vi "normal.vi"(3 "Settings":T1={"Horizontal Conf."={"Min. Sample rate"=0.0, "Reference position"=0.0, "Record Length"=0}, "Channel A"={"Enable"=FALSE, "Vertical coupling"=0, "Vertical range"=0.0, "Vertical offset"=0.0, "Probe attenuation"=1.0}, "Channel B"={"Enable"=FALSE, "Vertical coupling"=0, "Vertical range"=0.0, "Vertical offset"=0.0, "Probe attenuation"=1.0}, "Trigger"={"Source"=enum."channel 1", "Slope"=enum."Positive", "Coupling"=enum."AC", "Level"=0.0, "Holdoff"=0.0, "Delay"=0.0, "Timeout"=0.0, "Mode"=enum."Normal"}, "Measurements"={"Measurement 1, Channel"=enum."Channel 1", "Measurement 1, Selection"=enum."", "Measurement 2, Channel"=enum."Channel 1", "Measurement 2,  Selection"=enum."", "Measurement 3, Channel"=enum."Channel 1", "Measurement 3, Selection 3"=enum.""}}, 4 "error in":errorcluster caption="Error in" {"code" format="%.0x"}, 5 "instrument handle in":refnum<k15>) -> (0 "error out":errorcluster caption="Error out" {"code" format="%.0x"}, 1 "Adjusted Trigger Level":dbl, 2 "instrument handle out":refnum<k15>)   [LabVIEW 2011]
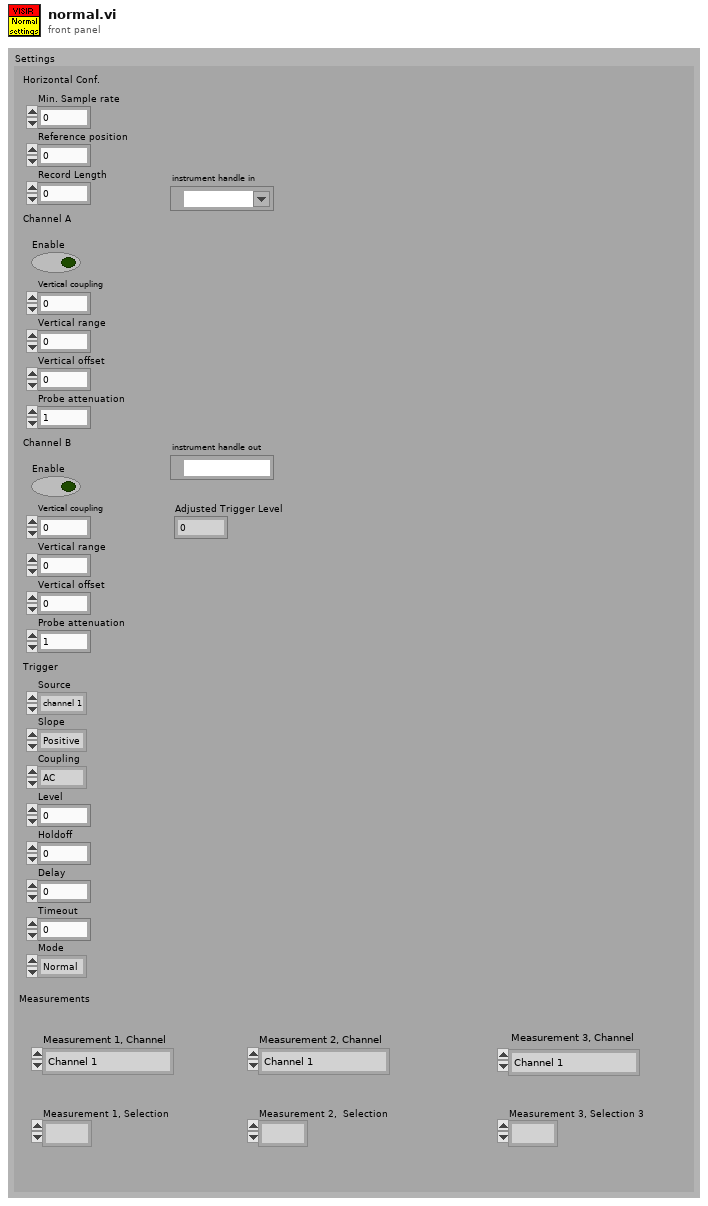
[diagram p1: front panel]
types:
  T1 = cluster{"Horizontal Conf.":cluster{"Min. Sample rate":dbl, "Reference position":dbl, "Record Length":i16}, "Channel A":cluster{"Enable":bool, "Vertical coupling":i32, "Vertical range":dbl, "Vertical offset":dbl, "Probe attenuation":dbl}, "Channel B":cluster{"Enable":bool, "Vertical coupling":i32, "Vertical range":dbl, "Vertical offset":dbl, "Probe attenuation":dbl}, "Trigger":cluster{"Source":enum8{"channel 1", "channel 2", "Imediate", "External trigger"}, "Slope":enum8{"Positive", "Negative"}, "Coupling":enum8{"AC", "DC"}, "Level":dbl, "Holdoff":dbl, "Delay":dbl, "Timeout":dbl, "Mode":enum8{"Normal", "Auto", "Auto Level"}}, "Measurements":cluster{"Measurement 1, Channel":enum8{"Channel 1", "Channel 2", "Channel 3", "Channel 4"}, "Measurement 1, Selection":enum16{""}, "Measurement 2, Channel":enum8{"Channel 1", "Channel 2", "Channel 3", "Channel 4"}, "Measurement 2,  Selection":enum16{""}, "Measurement 3, Channel":enum8{"Channel 1", "Channel 2", "Channel 3", "Channel 4"}, "Measurement 3, Selection 3":enum16{""}}}
  T2 = cluster{"Min. Sample rate":dbl, "Reference position":dbl, "Record Length":i16}
  T3 = cluster{"Enable":bool, "Vertical coupling":i32, "Vertical range":dbl, "Vertical offset":dbl, "Probe attenuation":dbl}
  T4 = cluster{"Source":enum8{"channel 1", "channel 2", "Imediate", "External trigger"}, "Slope":enum8{"Positive", "Negative"}, "Coupling":enum8{"AC", "DC"}, "Level":dbl, "Holdoff":dbl, "Delay":dbl, "Timeout":dbl, "Mode":enum8{"Normal", "Auto", "Auto Level"}}
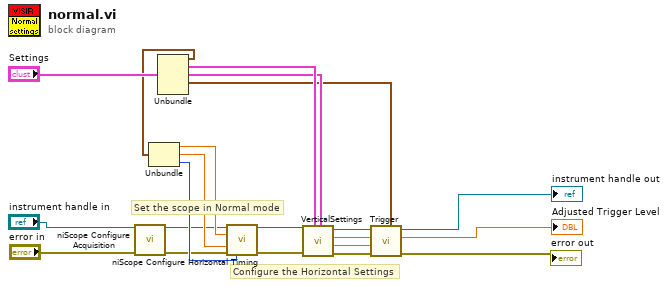
[diagram p0: block diagram]
diagram:
  # "Configure the Horizontal Settings"
  # "Set the scope in Normal mode"
  n1 = call <instrlib>:"niScope Configure Acquisition.vi"("instrument handle"="instrument handle in", "error in"="error in") -> ("instrument handle out"=w7:refnum<k15>, "error out"=w5:errorcluster)  [unwired: 12 in]
  n2 = Unbundle("Settings") -> ("Horizontal Conf."=w8:T2, "Channel A"=w19:T3, "Channel B"=w18:T3, "Trigger"=w17:T4)  [unwired: 1 out]
  n3 = Unbundle(w8) -> ("Min. Sample rate"=w11:dbl, "Reference position"=w10:dbl, "Record Length"=w9:i16)
  n4 = call <instrlib>:"niScope Configure Horizontal Timing.vi"("instrument handle"=w7, "min sample rate"=w11, "reference position"=w10, "error in"=w5, "min record length"=w9) -> ("instrument handle out"=w6:refnum<k15>, "error out"=w4:errorcluster)  [unwired: 9 in]
  n5 = call "VerticalSettings.vi"("Channel B"=w18, "Channel A"=w19, "error in"=w4, "instrument handle"=w6) -> ("error out"=w21:errorcluster, "Vertical range Channel B"=w2:dbl, "Vertical range Channel A"=w3:dbl, "instrument handle out"=w20:refnum<k15>)  [unwired: 4 in]
  n6 = call "Trigger.vi"("Trigger Settings"=w17, "error in"=w21, "Vertical range Channel B"=w2, "Vertical range Channel A"=w3, "instrument handle"=w20) -> ("error out"=→"error out":errorcluster, "Trigger Level"=→"Adjusted Trigger Level":dbl, "instrument handle"=→"instrument handle out":refnum<k15>)  [unwired: 4 in]
